vi "STM Listen for New Connections.vi"(8 "error in (no error)":errorcluster, 11 "State Variables":T1) -> (0 "error out":errorcluster)   [LabVIEW 2013, in "Control Addon Engine.lvlib" / "STM.lvlib"]
uses:
  STM.lvlib
  Inline Async API/Controls/Engine State Variables.ctl
  Stop FG/Stop Global Ref.ctl
  STM Comm Lookup Table_Ref.ctl
  Stop FG/Stop Global Commands.ctl
  <userlib>/STM/TCP/stm_TCP Read Options.ctl
  <userlib>/STM/Connection Manager/TCP/stm_TCPConnectionMethod.ctl
  <userlib>/STM/Connection Manager/TCP/stm_TCPConnectionProperties.ctl
  <userlib>/STM/TCP/STM Read Meta Data (TCP Ref).vi
  <vilib>/NI Veristand/Custom Device Tools/Custom Device Utility Library/Custom Device Utility Library.lvlib
  Stop FG/Stop FG.lvlib
  Error Handling API/Error Handling API.lvlib
  Inline Async API/Inline Async API.lvlib
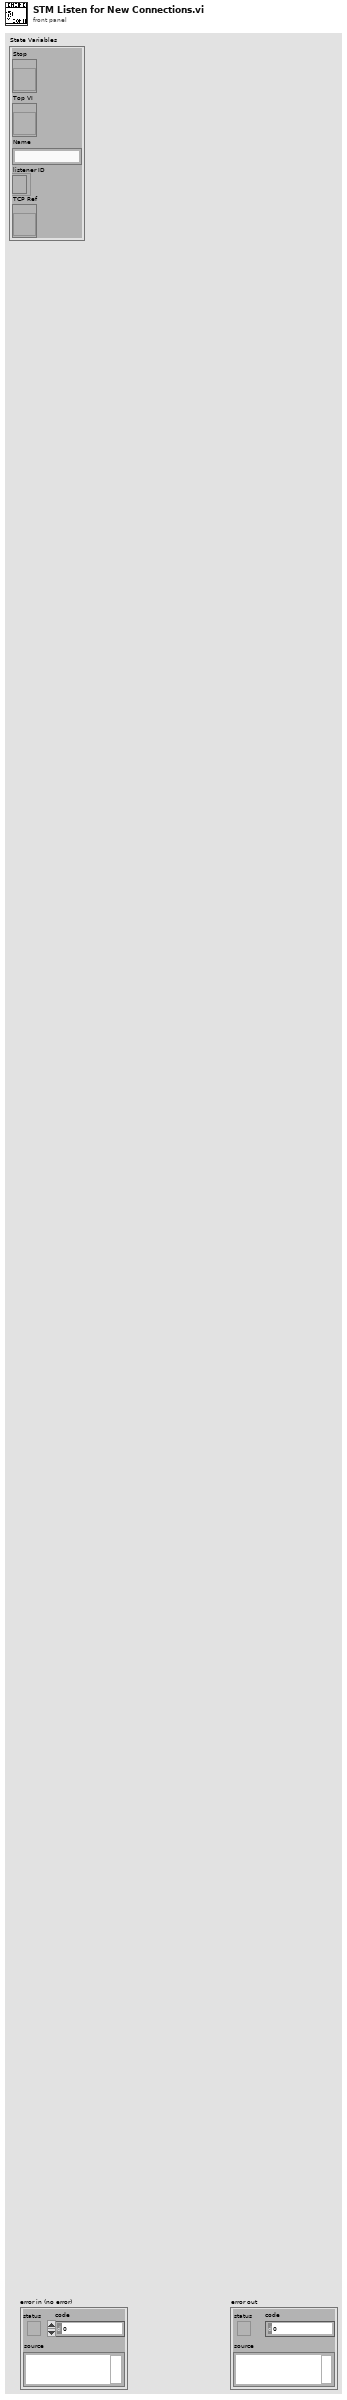
[diagram p1: front panel]
types:
  T1 = typedef "Control Addon Engine.lvlib/Inline Async API.lvlib/Engine State Variables.ctl" = cluster{"Stop":T2, "Top VI":refnum<vi>, "Name":string, "listener ID":refnum<k5>, "TCP Ref":T3}
  T2 = typedef "Control Addon Engine.lvlib/Stop FG.lvlib/Stop Global Ref.ctl" = refnum<vi>
  T3 = typedef "Control Addon Engine.lvlib/STM.lvlib/STM Comm Lookup Table_Ref.ctl" = refnum<vi>
  T4 = typedef "Control Addon Engine.lvlib/Stop FG.lvlib/Stop Global Commands.ctl" = enum16{"Write", "Read", "Reset"}
  T5 = typedef "stm_TCP Read Options.ctl" = cluster{"Ignore Timeout Error":bool, "timeout ms (1000)":i32}
  T6 = typedef "stm_TCPConnectionProperties.ctl" = cluster{"Name":string, "Address":string, "Custom":string}
  T7 = typedef "stm_TCPConnectionMethod.ctl" = enum16{"Initialize", "Add Connection", "Set Properties", "Get Connection(s)", "Remove Connection", "Remove All Connections", "Get Connection Count"}
  T8 = typedef "stm_TCP Connection Info.ctl" = cluster{"connection ID":refnum<k5>, "Meta data":T9[]}
  T9 = typedef "stm_MetaDataElement.ctl" = string
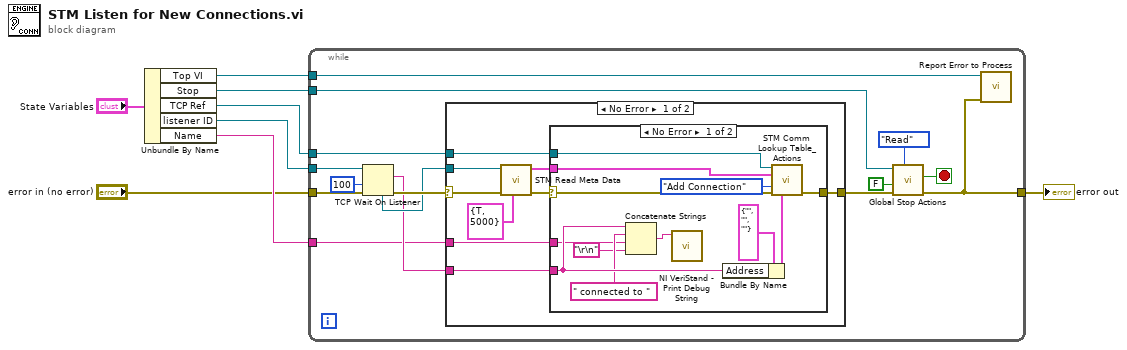
[diagram p0: block diagram]
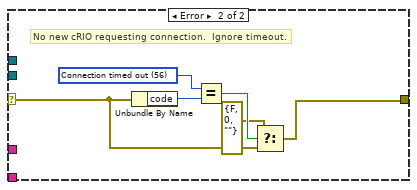
[diagram p3: hidden frame]
diagram:
  n1 = Unbundle By Name("State Variables") -> ("Top VI"=w7:refnum<vi>, "Stop"=w6:T2, "TCP Ref"=w5:T3, "listener ID"=w4:refnum<k5>, "Name"=w8:string)
  n2 = while {
    tunnel: "error in (no error)" -> [w23]
    tunnel: w4 -> [w22]
    tunnel: w6 -> [w15]
    tunnel: [w12] -> w2
    tunnel: w5 -> [w13]
    tunnel: w8 -> [w11]
    tunnel: w7 -> [w10]
    stop <- w17 stop-if-true
    n3 = TCP Wait On Listener(8:w23, 9:100 ("timeout ms (wait forever: -1)"), 11:w22) -> (0:w20:errorcluster, 2:w18:string, 4:w19:refnum<k5>)  [unwired: 1 in, 2 out]
    n4 = case shown="No Error" w20 {
      selector: w20 -> [w32 w48]
      tunnel: w19 -> [w31 _]
      tunnel: [w29 w47] -> w16
      tunnel: w18 -> [w26 _]
      tunnel: w13 -> [w28 _]
      tunnel: w11 -> [w25 _]
      frame No Error {
        n5 = call-poly <userlib>:"STM Read Meta Data.vi"("Options"=T5 {"Ignore Timeout Error"=TRUE, "timeout ms (1000)"=5000}, "error in"=w32, "connection ID"=w31) -> ("error out"=w27:errorcluster, "Connection Info Out"=w30:T8)  [unwired: 6 in, 1 out]
        n6 = case shown="No Error" w27 {
          selector: w27 -> [w41 w45]
          tunnel: w26 -> [w39 _]
          tunnel: w30 -> [w44 _]
          tunnel: [w43 w45] -> w29
          tunnel: w28 -> [w42 _]
          tunnel: w25 -> [w37 _]
          frame No Error {
            n7 = Concatenate Strings(w39, " connected to " ("string"), w37, "\r\n") -> (w40:string)
            n8 = call <vilib>:"NI VeriStand - Print Debug String.vi"("Message"=w40) -> ()  [unwired: 10 in, 1 out]
            n9 = Bundle By Name(cluster=T6 {"Name"="", "Address"="", "Custom"=""} ("Properties out"), "Address"=w39) -> (w34:T6)
            n10 = call "STM Comm Lookup Table_Actions.vi"("vi reference"=w42, "Connection In"=w44, "Method"=stm_TCPConnectionMethod."Add Connection", "error in (no error)"=w41, "Properties out"=w34) -> ("error out"=w43:errorcluster)  [unwired: 4 in, 6 out]
          }
          frame Error {
          }
        }
      }
      frame Error {
        w49 = 56 items=["No Error", "Argument Error", "Memory Full", "Out of Zone", "End of File", "File Already Open", "Generic File IO Error", "File Not Found", "File Permission Error", "Disk Full", "Duplicate Path", "Too Many Files Open", "Not Enabled", "Resource File Not Found", "Cannot Add Resource", "Resource Not Found", "Image Not Found", "Image Memory Error", "Pen Does Not Exist", "Config Bad Type", "Config Token Not Found", "Config Parse Error", "Config Memory Error", "Bad External Code Format", "Bad External Code Offset", "External Code Not Present", "Null Window", "Destroy Window Mixup", "Null Menu", "Print Aborted", "Bad Print Record", "Print Driver Error", "Windows Error During Print", "Memory Error During Print", "Print Dialog Error", "Generic Print Error", "Invalid Device Refnum", "Device Not Found", "Device Parameter Error", "Device Unit Error", "Can't Open Device", "Device Call Aborted", "Generic Error", "Cancelled By User", "Object ID Too Low", "Object ID Too High", "Object Not In Heap", "Unknown Heap", "Bad DefProc ID", "DefProc Not In Table", "Message Out Of Range", "Null Method", "Unknown Message", "Manager Call Not Supported", "Bad address", "Connection In progress", "Connection timed out", "Connection is already in progress", "Network attribute not supported", "Network error", "Address in use", "System out of memory", "Connection aborted", "Connection refused", "Connection is not connected", "Connection is already connected", "Connection closed", "Initialize error (interapplication manager)", "Bad occurrence", "Wait on unbound occurrence handler", "Occurrence queue overflow", "Bad path", "Semaphore not signaled", "Unrecognized type (interapplication manager)"] ("1st Error to Convert")
        # "No new cRIO requesting connection.  Ignore timeout."
        n11 = Unbundle By Name(w48) -> ("code"=w50:i32)
        n12 = Equal?(x=w49, y=w50) -> (x = y?=w51:bool)
        n13 = Select(t=errorcluster {"status"=FALSE, "code"=0, "source"=""} ("error in (no error)"), s=w51, f=w48) -> (s? t:f=w47:errorcluster)
      }
    }
    n14 = call "Global Stop Actions.vi"("Command"=Stop_Global_Commands."Read", "error in (no error)"=w16, "Stop on Error?"=FALSE, "vi reference"=w15) -> ("error out"=w12:errorcluster, "Latched Stop"=w17:bool)  [unwired: 5 in, 1 out]
    n15 = call "Report Error to Process.vi"("Error"=w12, "This VI"=w10) -> ()  [unwired: 10 in]
  }
  "error out" <- w2
